vi "C++ Syntax Highlighter.vi"(8 "Error In":errorcluster, 11 "control/indicator refnum in":refnum<vi>) -> (0 "Error Out":errorcluster)   [LabVIEW 2014]
doc: "Highlight C/C++ by controls on front panel inside this VI. If you want to create other color scheme, please copy it and store values as defaults.\n\nBased on: https://forums.ni.com/t5/Example-Programs/Finding-and-Highlighting-or-Coloring-a-Word-in-a-String-Control/ta-p/3508601"
panel:
  in  "colours":u32[](array[colorbox])=[0, 0, 11796564, 16860, 11796564, 16860, 16860, 16748288, 16860, 0, 9868950, 1985280, 10455040, 36351, 16860, 3071, 16748288, 16860, 0, 0, 0, 16860, 1985280, 0, 0, 0, 0, 16711680]
  in  "Bold?":bool[](array[boolean])=[TRUE, FALSE, FALSE, FALSE, FALSE, FALSE, FALSE, FALSE, FALSE, FALSE, TRUE, TRUE, FALSE, FALSE, FALSE, FALSE, FALSE, TRUE, TRUE, TRUE, TRUE, FALSE, FALSE, TRUE, TRUE, TRUE, TRUE, TRUE]
  in  "dictionary":string[](array[string])=["if", "shift", "String", "LVSubVI_", "void", "(", ")", "float", "int", "print", "return", "bool", "shiftRegister_", "unsigned char", "unsigned long", "iteratorUID_", "Serial", "case", "true", "false", "vector", "long", "File", "for", "switch", "feedbackNode_", "break;", "/* Don't know how to translate class"]
  # "<--- to not color int word inside it :D"
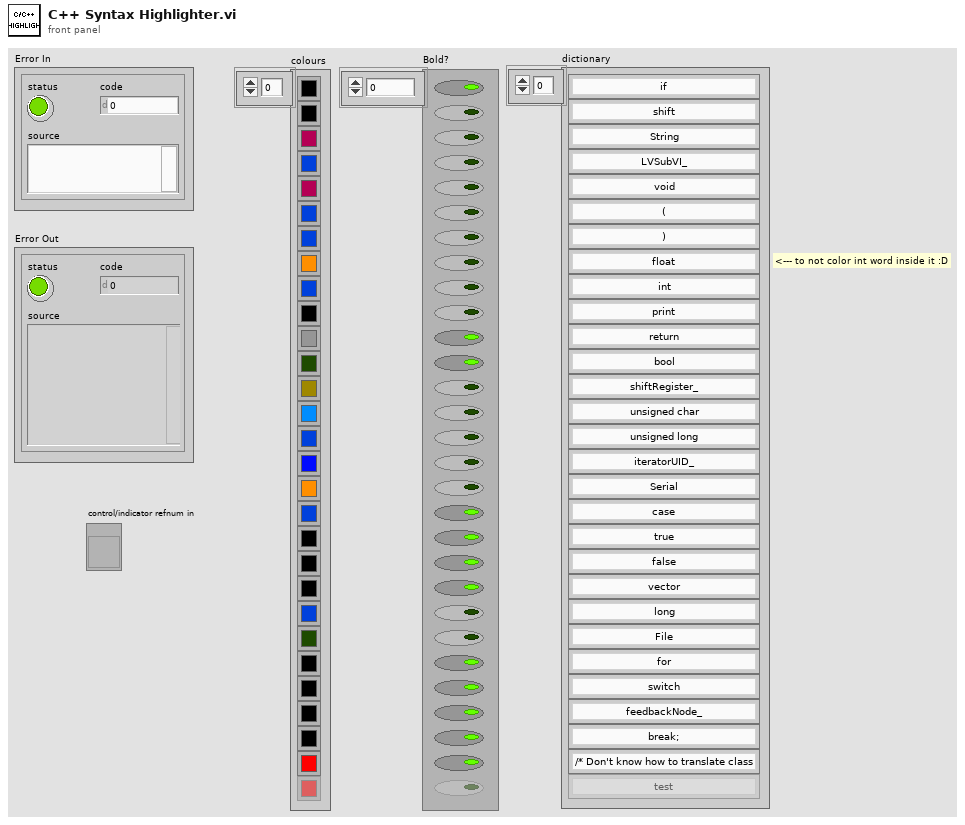
[diagram p1: front panel]
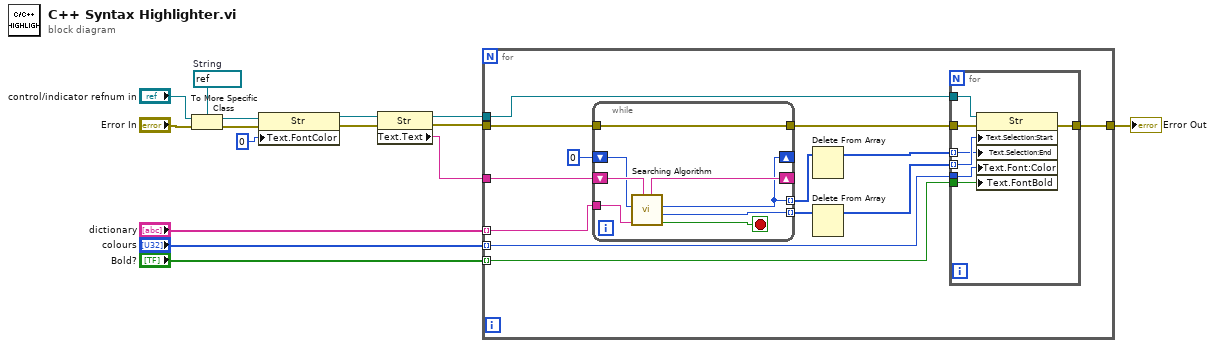
[diagram p0: block diagram]
diagram:
  w11 = refnum<vi> refnum  # String
  n1 = To More Specific Class(target class=w11, reference="control/indicator refnum in", error in="Error In") -> (specific class reference=w10:refnum<vi>, error out=w9:errorcluster)
  n2 = property class="Str"(reference=w10, error in=w9, "Text.FontColor"=u32 0 ("Text.Font:Color")) -> (reference out=w6:refnum<vi>, error out=w5:errorcluster)
  n3 = property class="Str"(reference=w6, error in=w5) -> (reference out=w3:refnum<vi>, error out=w4:errorcluster, "Text.Text"=w2:string)
  n4 = for {
    tunnel: w4 -> [w21]
    tunnel: [w23] -> w15
    tunnel: "dictionary" -> [w20] mode=indexing
    tunnel: "colours" -> [w19] mode=indexing
    tunnel: w3 -> [w18]
    tunnel: w2 -> [w17]
    tunnel: "Bold?" -> [w16] mode=indexing
    n5 = while {
      tunnel: [w38] -> w28 mode=indexing
      tunnel: [w39] -> w27 mode=indexing
      shift-right: [w41] -> _
      shift-left: w17 -> [w43]
      shift-right: [w38] -> _
      shift-left: 0 ("Numeric 2") -> [w40]
      tunnel: w20 -> [w37]
      tunnel: [w36] -> w22
      tunnel: w21 -> [w36]
      stop <- w42 stop-if-true
      n6 = call "Searching Algorithm.vi"("Input String"=w43, "Find"=w37, "Start Index"=w40) -> ("Done?"=w42:bool, "Start of Find"=w39:u32, "End of Find"=w38:u32, "After Match"=w41:string)  [unwired: 5 in]
    }
    n7 = Delete From Array "Delete From Array"(array=w28) -> (array with subset deleted=w25:u32[])  [unwired: 2 in, 1 out]
    n8 = Delete From Array "Delete From Array"(array=w27) -> (array with subset deleted=w26:u32[])  [unwired: 2 in, 1 out]
    n9 = for {
      tunnel: w26 -> [w35] mode=indexing
      tunnel: w25 -> [w34] mode=indexing
      tunnel: [w32] -> w23
      tunnel: w22 -> [w33]
      tunnel: w19 -> [w31]
      tunnel: w18 -> [w30]
      tunnel: w16 -> [w29]
      n10 = property on="Property Node" class="Str"(reference=w30, error in=w33, "Text.Selection:Start"=w35, "Text.Selection:End"=w34, "Text.Font:Color"=w31, "Text.FontBold"=w29) -> (error out=w32:errorcluster)  [unwired: 1 out]
    }
  }
  "Error Out" <- w15
